vi "Main.vi"() -> ()   [LabVIEW 2017]
uses:
  <vilib>/addons/InsightCM/MessageBus/MessageLibrary/SysCfgDeployer/controls/SysCfgDeployPackageRequestBody.ctl
  subVIs/States.ctl
  <vilib>/addons/InsightCM/MessageBus/MessageService/IcmMessageService.lvclass
panel:
  out "path":path
  out "State":T1=enum."CheckForOnlineDevices"
  out "BatchDevicesToUpdate":T2[](array[typedef])
  out "error out":errorcluster
  in  "stop":bool
  in  "DeployImage":bool
  out "Online Devices":i32
  out "Devices To Update - all info":T2[](array[typedef])
  out "Devices To Update":string[](array[string])
  out "SubsetForBatchDeploy":T2[](array[typedef])
  out "Status":string
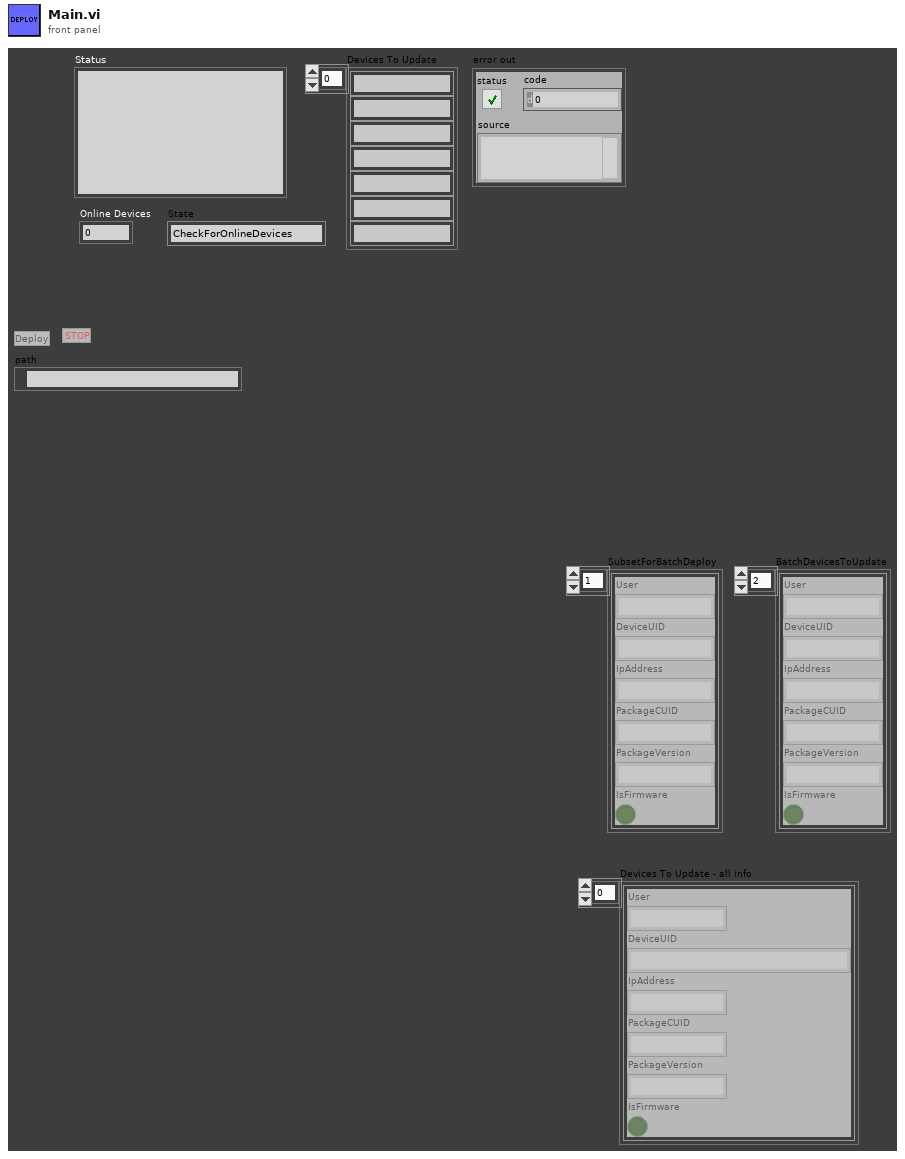
[diagram p1: front panel]
types:
  T1 = typedef "States.ctl" = enum16{"Deploy", "Wait", "CheckForOnlineDevices", "Init", "DeviceSubset", "ResetSMS", "Check", "Report", "Reset", "ResetConn"}
  T2 = typedef "SysCfgDeployPackageRequestBody.ctl" = cluster{"User":string, "DeviceUID":string, "IpAddress":string, "PackageCUID":string, "PackageVersion":string, "IsFirmware":bool}
  T3 = enum8{"Enabled", "Disabled", "Disabled and Grayed Out"}
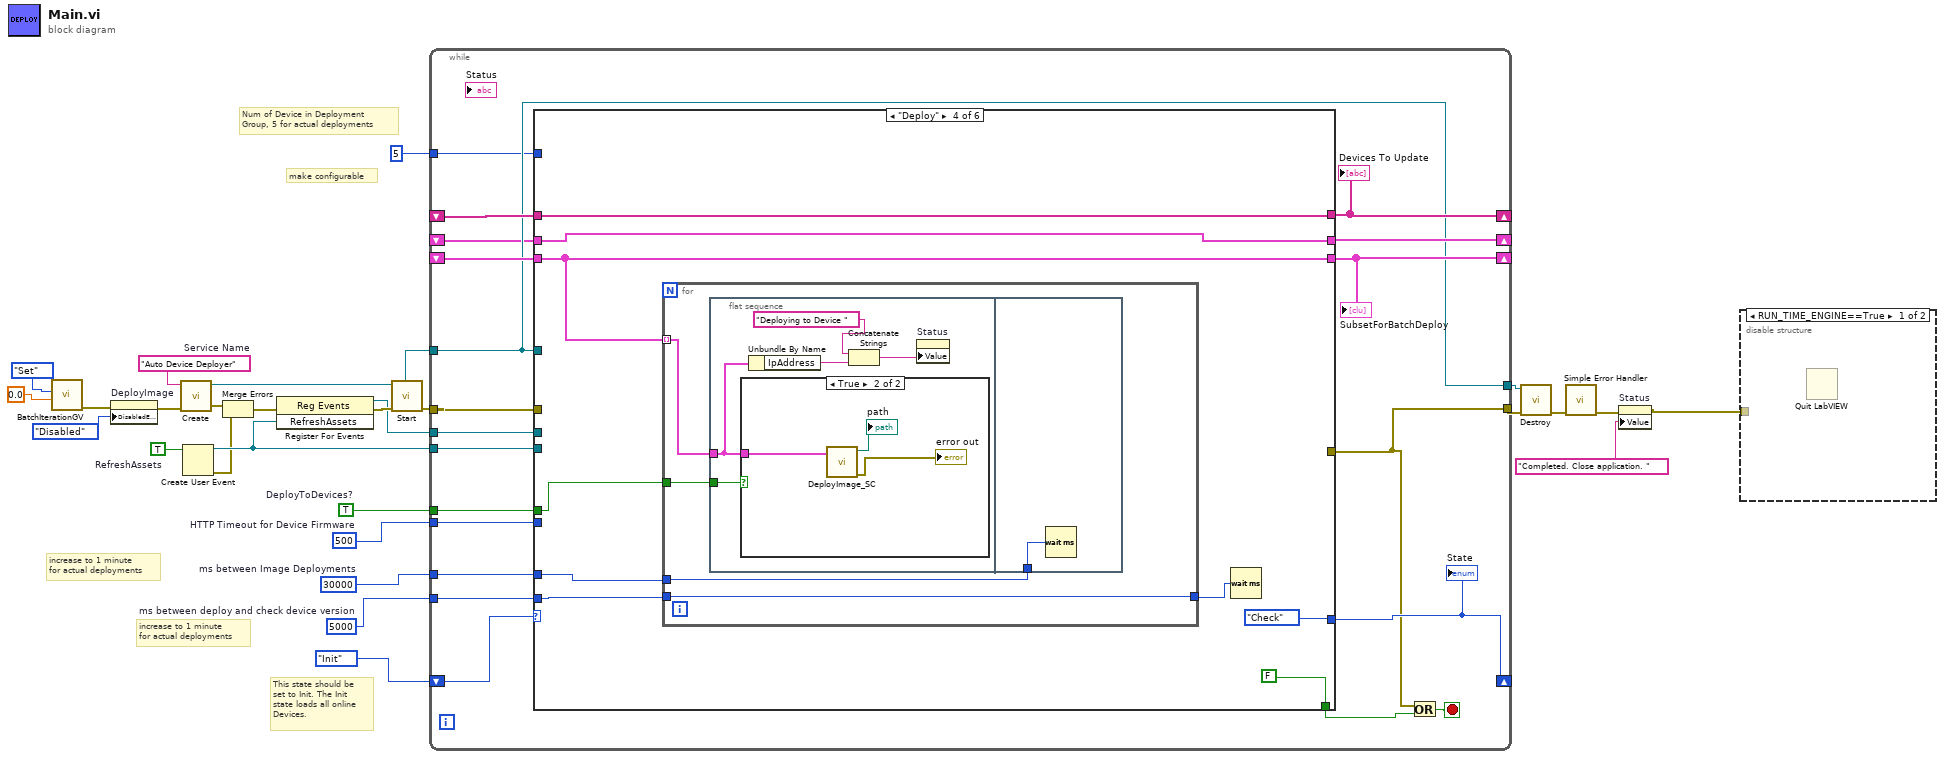
[diagram p0: block diagram]
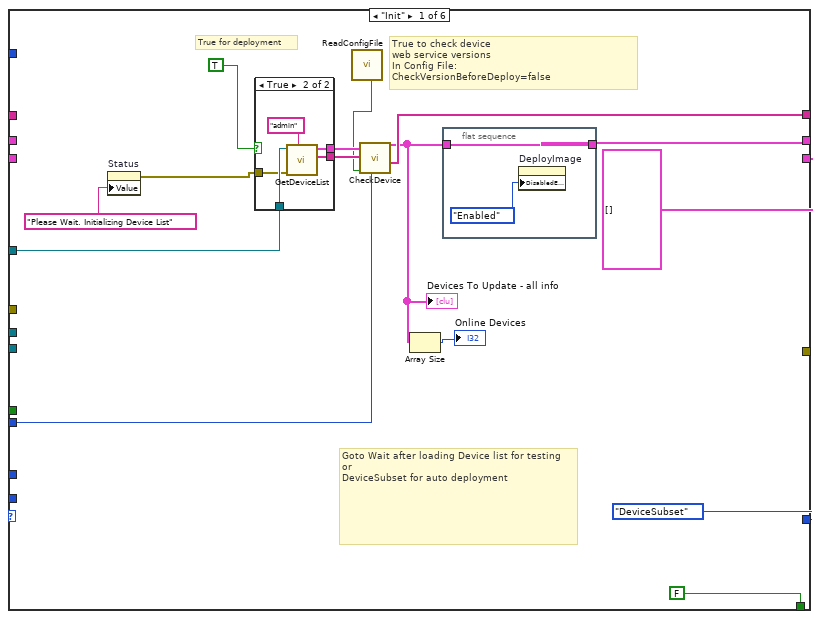
[diagram p3: hidden frame]
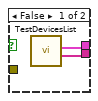
[diagram p4: hidden frame]
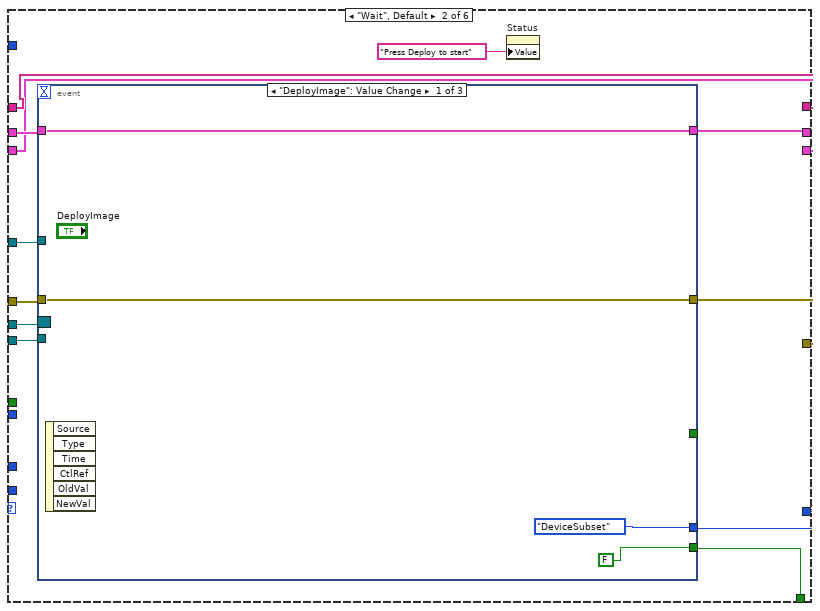
[diagram p5: hidden frame]
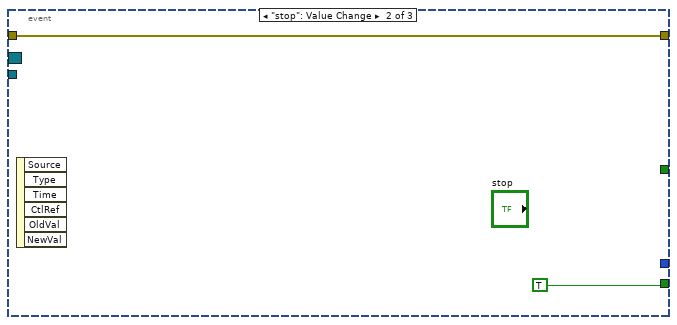
[diagram p6: hidden frame]
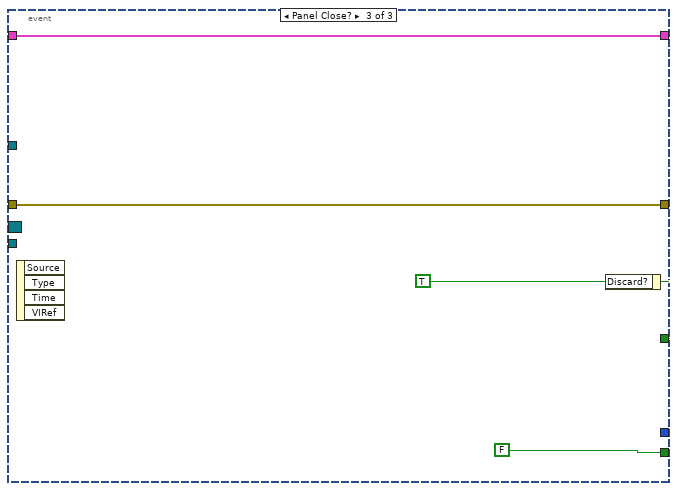
[diagram p7: hidden frame]
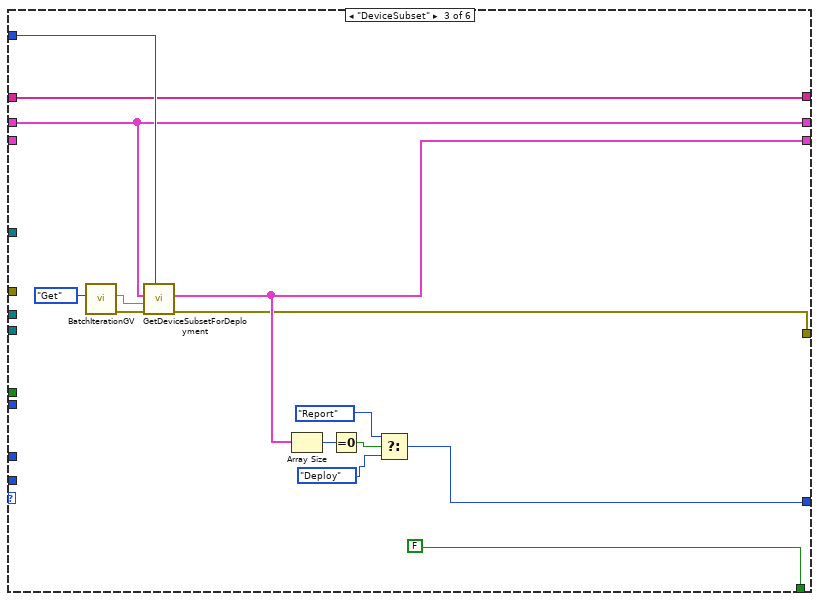
[diagram p8: hidden frame]
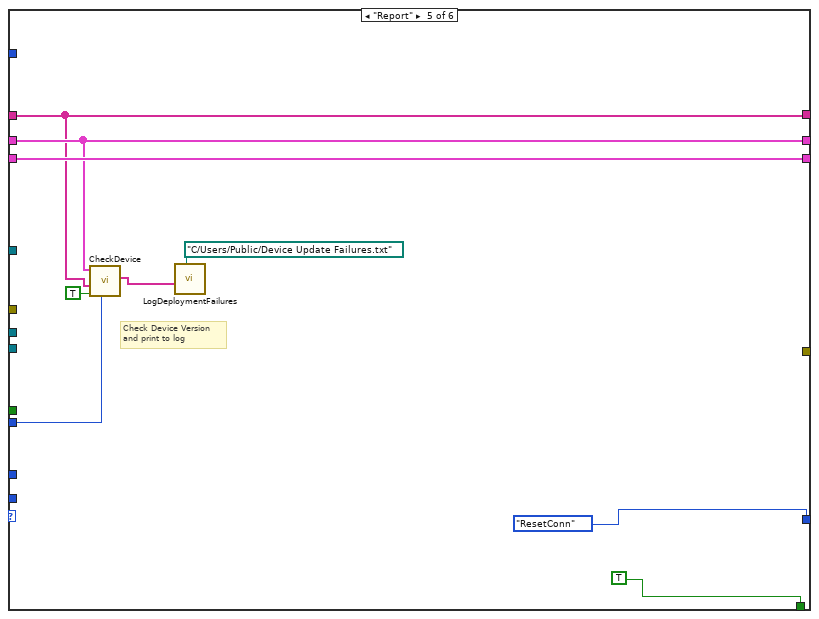
[diagram p10: hidden frame]
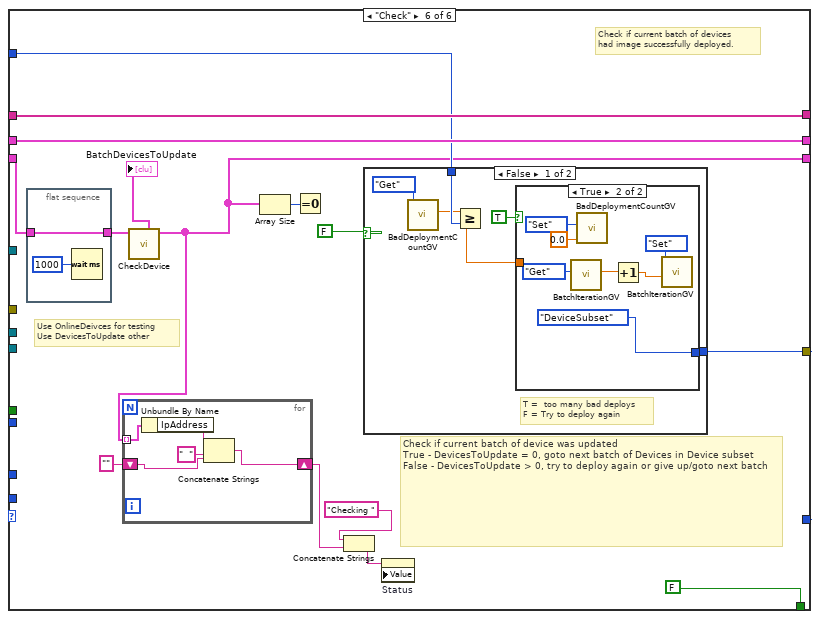
[diagram p11: hidden frame]
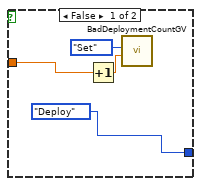
[diagram p12: hidden frame]
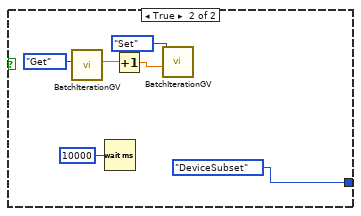
[diagram p13: hidden frame]
diagram:
  w7 = u32 5000  # ms between deploy and check device version
  w10 = TRUE  # DeployToDevices?
  w14 = 500  # HTTP Timeout for Device Firmware
  w16 = u32 30000  # ms between Image Deployments
  w25 = TRUE  # RefreshAssets
  w28 = "Auto Device Deployer"  # Service Name
  # "make configurable"
  # "increase to 1 minute\nfor actual deployments"
  # "increase to 1 minute\nfor actual deployments"
  # "This state should be \nset to Init. The Init \nstate loads all online\nDevices."
  # "Num of Device in Deployment\nGroup, 5 for actual deployments"
  n1 = call "BatchIterationGV.vi"("SetIteration"=0.0, "GetOrSet"=enum16{"Get", "Set"}."Set") -> ("error out"=w4:errorcluster)  [unwired: 7 in, 2 out]
  n2 = property on="DeployImage" class="Bool"(error in=w4, "DisabledEnum"=T3."Disabled" ("Disabled")) -> (error out=w9:errorcluster)  [unwired: 1 in, 1 out]
  n3 = call <vilib>:"Create.vi"("error in (no error)"=w9, "service name"=w28) -> ("error out"=w21:errorcluster, "service out"=w27:refnum<class "IcmMessageService.lvclass">)  [unwired: 8 in]
  n4 = Create User Event(user event datatype=w25) -> (user event=w22:refnum<user-event>, error out=w20:errorcluster)  [unwired: 1 in]
  n5 = Merge Errors(w21, w20) -> (w19:errorcluster)
  n6 = register-events(error in=w19, w22) -> (reference out=w23:refnum<event-registration>, error out=w24:errorcluster)  [unwired: 1 in]
  n7 = call <vilib>:"Start.vi"("error in (no error)"=w24, "service in"=w27) -> ("error out"=w26:errorcluster, "service out"=w18:refnum<class "IcmMessageService.lvclass">)  [unwired: 8 in]
  n8 = while {
    tunnel: w18 -> [w36]
    tunnel: w26 -> [w48]
    tunnel: w23 -> [w47]
    tunnel: w22 -> [w46]
    shift-right: [w45] -> _
    shift-left: _ -> [w30]
    shift-right: [w43] -> _
    shift-left: States."Init" -> [w44]
    shift-right: [w42] -> _
    shift-left: _ -> [w41]
    shift-right: [w40] -> _
    shift-left: _ -> [w39]
    tunnel: 5 ("num") -> [w29]
    tunnel: w16 -> [w38]
    tunnel: [w33] -> w13
    tunnel: w14 -> [w37]
    tunnel: [w36] -> w11
    tunnel: w10 -> [w35]
    tunnel: w7 -> [w31]
    stop <- w34 stop-if-true
    n9 = case shown="\"Deploy\"" w44 {
      tunnel: w48 -> [_ w84 _ _ _ _]
      tunnel: [_ w83 w98 _ _ _] -> w33
      tunnel: w47 -> [_ w82 _ _ _ _]
      tunnel: w46 -> [_ w81 _ _ _ _]
      tunnel: w30 -> [_ w80 w97 w117 w137 w153]
      tunnel: w36 -> [w63 w79 _ _ _ _]
      tunnel: [w57 w78 w97 w117 w137 w153] -> w45
      tunnel: [States."DeviceSubset" w77 w101 States."Check" States."ResetConn" w150] -> w43
      tunnel: [w61 w76 w107 w116 w136 w154] -> w42
      tunnel: w41 -> [_ w76 w107 w116 w136 w154]
      tunnel: [T2[] [] ("subarray") w75 w102 w115 w139 w145] -> w40
      tunnel: w39 -> [_ w75 _ w115 w139 w147]
      tunnel: w29 -> [_ _ w108 _ _ w151]
      tunnel: w38 -> [_ _ _ w114 _ _]
      tunnel: w37 -> [w60 _ _ _ w135 _]
      tunnel: w35 -> [_ _ _ w112 _ _]
      tunnel: [FALSE w73 FALSE FALSE TRUE ("Discard?") FALSE] -> w32
      tunnel: w31 -> [_ _ _ w109 _ _]
      frame "Init" {
        # "True to check device\nweb service versions\nIn Config File:\nCheckVersionBeforeDeploy=false"
        # "True for deployment"
        # "Goto Wait after loading Device list for testing \nor\nDeviceSubset for auto deployment"
        n10 = property on="Status" class="Str"("Value"="Please Wait. Initializing Device List" ("Message")) -> (error out=w51:errorcluster)  [unwired: 2 in, 1 out]
        n11 = case shown="True" TRUE {
          tunnel: w63 -> [_ w70]
          tunnel: w51 -> [_ w69]
          tunnel: [w65 w67] -> w54
          tunnel: [w64 w66] -> w53
          frame False {
            n12 = call "TestDevicesList.vi"() -> ("Names"=w64:string[], "Array"=w65:T2[])  [unwired: 10 in]
          }
          frame True {
            n13 = call "GetDeviceList.vi"("User"="admin", "error in (no error)"=w69, "IcmMessageService in"=w70) -> ("DeviceNames"=w66:string[], "DeviceList"=w67:T2[])  [unwired: 6 in, 1 out]
          }
        }
        n14 = call "ReadConfigFile.vi"() -> ("CheckVersionBeforeDeploy"=w49:bool)  [unwired: 6 in, 5 out]
        n15 = call "CheckDevice.vi"("timeout (10000)"=w60, "CheckVersion"=w49, "DevicesNames"=w53, "DeviceList"=w54) -> ("DevicesToUpdateNames"=w61:string[], "DevicesToUpdate"=w56:T2[])  [unwired: 2 in, 4 out]
        "Devices To Update - all info" <- w56
        n16 = Array Size(array=w56) -> (size(s)=→"Online Devices":i32)
        n17 = flat-sequence {
          tunnel: [w72] -> w57
          tunnel: w56 -> [w72]
          frame #0 {
            n18 = property on="DeployImage" class="Bool"("DisabledEnum"=T3."Enabled" ("Disabled")) -> ()  [unwired: 2 in, 2 out]
          }
        }
      }
      frame "Wait", Default {
        n19 = event shown="[0] \"DeployImage\": Value Change" {
          selector: w82 -> [_ _ _]
          dyn-events: _ -> [_ _ _]
          timeout: _ -> [_ _ _]
          tunnel: w84 -> [w88 w90 w93]
          tunnel: w79 -> [_ _ _]
          tunnel: [_ _ w94] -> _
          tunnel: [w88 w90 w93] -> w83
          tunnel: w81 -> [_ _ _]
          tunnel: w80 -> [w87 _ w92]
          tunnel: [w87 _ w92] -> w78
          tunnel: [States."DeviceSubset" _ _] -> w77
          tunnel: [FALSE TRUE FALSE] -> w73
          event "DeployImage": Value Change {
            n20 = event-data() -> ()  [unwired: 1 in, 6 out]
          }
          event "stop": Value Change {
            n21 = event-data() -> ()  [unwired: 1 in, 6 out]
          }
          event Panel Close? {
            w94 = TRUE ("Discard?")
            n22 = event-data() -> ()  [unwired: 1 in, 4 out]
            n23 = event-data("Discard?"=w94) -> ()  [unwired: 1 in, 1 out]
          }
        }
        n24 = property on="Status" class="Str"("Value"="Press Deploy to start" ("Message")) -> ()  [unwired: 2 in, 2 out]
      }
      frame "DeviceSubset" {
        n25 = call "BatchIterationGV.vi"("GetOrSet"=enum16{"Get", "Set"}."Get") -> ("error out"=w105:errorcluster, "Iteration"=w106:dbl)  [unwired: 8 in, 1 out]
        n26 = call "GetDeviceSubsetForDeployment.vi"("num"=w108, "error in (no error)"=w105, "i"=w106, "DeviceList"=w97) -> ("Error Out"=w98:errorcluster, "subarray"=w102:T2[])  [unwired: 6 in]
        n27 = Array Size(array=w102) -> (size(s)=w103:i32)
        n28 = Equal To 0?(x=w103) -> (x = 0?=w96:bool)
        n29 = Select(t=States."Report", s=w96, f=States."Deploy") -> (s? t:f=w101:T1)
      }
      frame "Deploy" {
        n30 = for {
          tunnel: w115 -> [w119] mode=indexing
          tunnel: w114 -> [w121]
          tunnel: w112 -> [w120]
          tunnel: [w118] -> w110
          tunnel: w109 -> [w118]
          n31 = flat-sequence {
            tunnel: w119 -> [w122]
            tunnel: w120 -> [w126]
            tunnel: w121 -> [w130]
            frame #0 {
              n32 = case shown="True" w126 {
                tunnel: w122 -> [_ w129]
                frame False {
                }
                frame True {
                  n33 = call "DeployImage_SC.vi"("SysCfgDeployRequest"=w129) -> ("error out"=→"error out":errorcluster, "path"=→"path":path)  [unwired: 9 in]
                }
              }
              n34 = Unbundle By Name(w122) -> ("IpAddress"=w124:string)
              n35 = Concatenate Strings("Deploying to Device " ("Message"), w124) -> (w125:string)
              n36 = property on="Status" class="Str"("Value"=w125) -> ()  [unwired: 2 in, 2 out]
            }
            frame #1 {
              n37 = Wait (ms)(milliseconds to wait=w130) -> ()  [unwired: 1 out]
            }
          }
        }
        n38 = Wait (ms)(milliseconds to wait=w110) -> ()  [unwired: 1 out]
      }
      frame "Report" {
        # "Check Device Version\nand print to log"
        n39 = call "CheckDevice.vi"("timeout (10000)"=w135, "CheckVersion"=TRUE, "DevicesNames"=w136, "DeviceList"=w137) -> ("NotUpdatedDevicesNames"=w131:string[])  [unwired: 2 in, 5 out]
        n40 = call "LogDeploymentFailures.vi"("UpdatedDevices"=path "C:/Users/Public/Device Update Failures.txt", "Names"=w131) -> ()  [unwired: 10 in]
      }
      frame "Check" {
        # "Use OnlineDeivces for testing\nUse DevicesToUpdate other"
        # "Check if current batch of devices \nhad image successfully deployed."
        # "Check if current batch of device was updated\nTrue - DevicesToUpdate = 0, goto next batch of Devices in Device subset\nFalse - DevicesToUpdate > 0, try to deploy again or give up/goto next batch"
        n41 = flat-sequence {
          tunnel: w147 -> [w161]
          tunnel: [w161] -> w146
          frame #0 {
            n42 = Wait (ms)(milliseconds to wait=u32 1000) -> ()  [unwired: 1 out]
          }
        }
        n43 = call "CheckDevice.vi"("DeviceList"=w146) -> ("OnlineDevices"=w145:T2[], "DevicesToUpdate"=→"BatchDevicesToUpdate":T2[])  [unwired: 5 in, 4 out]
        n44 = for {
          tunnel: w145 -> [w159] mode=indexing
          shift-right: [w157] -> w144
          shift-left: "" -> [w156]
          n45 = Unbundle By Name(w159) -> ("IpAddress"=w158:string)
          n46 = Concatenate Strings(w158, "  " ("string"), w156) -> (w157:string)
        }
        n47 = Array Size(array=w145) -> (size(s)=w148:i32)
        n48 = Equal To 0?(x=w148) -> ()  [unwired: 1 out]
        n49 = Concatenate Strings("Checking " ("Status"), w144) -> (w142:string)
        n50 = case shown="False" FALSE {
          tunnel: w151 -> [w165 _]
          tunnel: [w163 States."DeviceSubset"] -> w150
          frame False {
            # "T =  too many bad deploys\nF = Try to deploy again"
            n51 = call "BadDeploymentCountGV.vi"("GetOrSet"=enum16{"Get", "Set"}."Get") -> ("BadDeployCount"=w164:dbl)  [unwired: 9 in, 1 out]
            n52 = Greater Or Equal?(x=w164, y=w165) -> ()  [unwired: 1 out]
            n53 = case shown="True" TRUE {
              tunnel: w164 -> [w168 _]
              tunnel: [States."Deploy" States."DeviceSubset"] -> w163
              frame False {
                n54 = Increment(x=w168) -> (x+1=w169:dbl)
                n55 = call "BadDeploymentCountGV.vi"("SetBadDeployments"=w169, "GetOrSet"=enum16{"Get", "Set"}."Set") -> ()  [unwired: 8 in, 2 out]
              }
              frame True {
                n56 = call "BatchIterationGV.vi"("GetOrSet"=enum16{"Get", "Set"}."Get") -> ("Iteration"=w174:dbl)  [unwired: 8 in, 2 out]
                n57 = call "BadDeploymentCountGV.vi"("SetBadDeployments"=0.0, "GetOrSet"=enum16{"Get", "Set"}."Set") -> ()  [unwired: 8 in, 2 out]
                n58 = Increment(x=w174) -> (x+1=w173:dbl)
                n59 = call "BatchIterationGV.vi"("SetIteration"=w173, "GetOrSet"=enum16{"Get", "Set"}."Set") -> ()  [unwired: 7 in, 3 out]
              }
            }
          }
          frame True {
            n60 = call "BatchIterationGV.vi"("GetOrSet"=enum16{"Get", "Set"}."Get") -> ("Iteration"=w182:dbl)  [unwired: 8 in, 2 out]
            n61 = Wait (ms)(milliseconds to wait=u32 10000) -> ()  [unwired: 1 out]
            n62 = Increment(x=w182) -> (x+1=w181:dbl)
            n63 = call "BatchIterationGV.vi"("SetIteration"=w181, "GetOrSet"=enum16{"Get", "Set"}."Set") -> ()  [unwired: 7 in, 3 out]
          }
        }
        n64 = property on="Status" class="Str"("Value"=w142) -> ()  [unwired: 2 in, 2 out]
      }
    }
    "Devices To Update" <- w42
    "SubsetForBatchDeploy" <- w40
    "State" <- w43
    n65 = Or(x=w33, y=w32) -> (x .or. y?=w34:bool)
  }
  n66 = call <vilib>:"Destroy.vi"("error in (no error)"=w13, "service in"=w11) -> ("error out"=w12:errorcluster)  [unwired: 9 in]
  n67 = call <vilib>:"Simple Error Handler.vi"("error in (no error)"=w12) -> ("error out"=w3:errorcluster)  [unwired: 4 in, 4 out]
  n68 = property on="Status" class="Str"(error in=w3, "Value"="Completed. Close application. " ("Status")) -> (error out=w2:errorcluster)  [unwired: 1 in, 1 out]
  n69 = disable-structure shown="RUN_TIME_ENGINE==True" {
    disable-tunnel: w2 -> [_ _]
    frame condition #0 {
      n70 = Quit LabVIEW() -> ()  [unwired: 1 in]
    }
    frame condition #1 (active) {
    }
  }
